vi "Enable Output.vi"(8 "error in (no error)":errorcluster, 9 "Enable?":bool, 10 "Output":T1, 11 "LINX-ExplorerHatPro in":refnum<class "LINX-ExplorerHatPro.lvclass">) -> (0 "error out":errorcluster, 3 "LINX-ExplorerHatPro out":refnum<class "LINX-ExplorerHatPro.lvclass">)   [LabVIEW 2020, in "LINX-ExplorerHatPro.lvclass"]
uses:
  LINX-ExplorerHatPro.lvclass
  GPIO/LINX GPIO.lvclass
  Output Pins.ctl
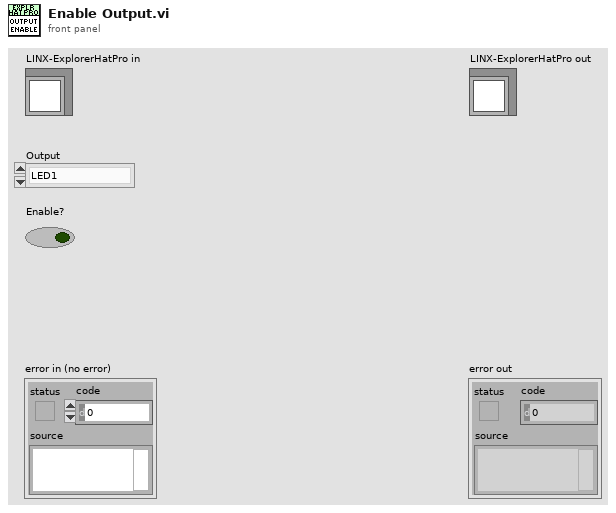
[diagram p1: front panel]
types:
  T1 = typedef "LINX-ExplorerHatPro.lvclass/Output Pins.ctl" = enum16{"LED1", "LED2", "LED3", "LED4", "OUTPUT1", "OUTPUT2", "OUTPUT3", "OUTPUT4"}
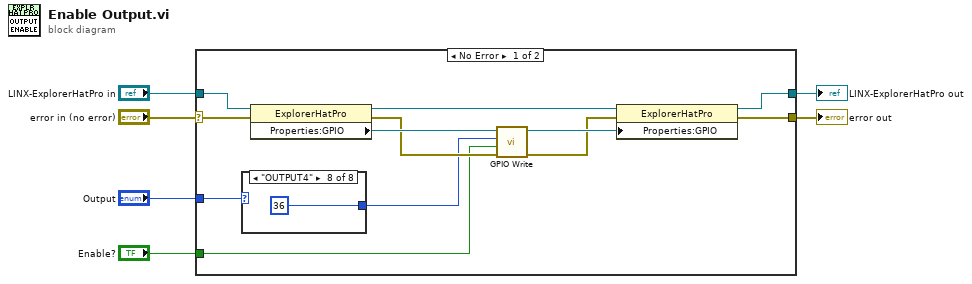
[diagram p0: block diagram]
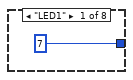
[diagram p2: hidden frame]
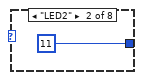
[diagram p3: hidden frame]
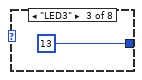
[diagram p4: hidden frame]
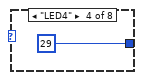
[diagram p5: hidden frame]
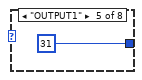
[diagram p6: hidden frame]
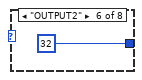
[diagram p7: hidden frame]
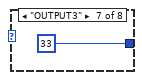
[diagram p8: hidden frame]
diagram:
  n1 = case shown="No Error" "error in (no error)" {
    selector: "error in (no error)" -> [w10 w28]
    tunnel: [w9 w28] -> w5
    tunnel: [w16 w27] -> w3
    tunnel: "LINX-ExplorerHatPro in" -> [w18 w27]
    tunnel: "Enable?" -> [w11 _]
    tunnel: "Output" -> [w8 _]
    frame No Error {
      n2 = case shown="\"OUTPUT4\"" w8 {
        tunnel: [u8 7 ("DO Channel") u8 11 ("DO Channel") u8 13 ("DO Channel") u8 29 ("DO Channel") u8 31 ("DO Channel") u8 32 ("DO Channel") u8 33 ("DO Channel") u8 36 ("DO Channel")] -> w7
        frame "LED1" {
        }
        frame "LED2" {
        }
        frame "LED3" {
        }
        frame "LED4" {
        }
        frame "OUTPUT1" {
        }
        frame "OUTPUT2" {
        }
        frame "OUTPUT3" {
        }
        frame "OUTPUT4" {
        }
      }
      n3 = property class="ExplorerHatPro"(reference=w18, error in=w10) -> (reference out=w17:refnum<class "LINX-ExplorerHatPro.lvclass">, error out=w14:errorcluster, "Properties:GPIO"=w15:refnum<class "LINX GPIO.lvclass">)
      n4 = call-dynamic "GPIO Write.vi"("error in (no error)"=w14, "Output Value"=w11, "DO Channel"=w7, "LINX GPIO in"=w15) -> ("error out"=w12:errorcluster, "LINX GPIO out"=w13:refnum<class "LINX GPIO.lvclass">)  [unwired: 6 in]
      n5 = property class="ExplorerHatPro"(reference=w17, error in=w12, "Properties:GPIO"=w13) -> (reference out=w16:refnum<class "LINX-ExplorerHatPro.lvclass">, error out=w9:errorcluster)
    }
    frame Error {
    }
  }
  "error out" <- w5
  "LINX-ExplorerHatPro out" <- w3
